vi "GetCntrlRefs.vi"(11 "CntrlRefs":T1) -> (3 "CntrlRefs":T1)   [LabVIEW 2018]
uses:
  CntrlRefs.ctl
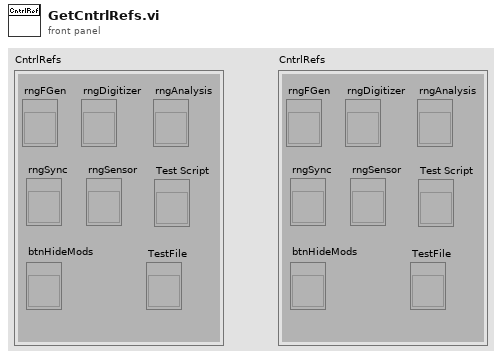
[diagram p1: front panel]
types:
  T1 = typedef "CntrlRefs.ctl" = cluster{"rngFGen":refnum<vi>, "rngDigitizer":refnum<vi>, "rngAnalysis":refnum<vi>, "rngSync":refnum<vi>, "btnHideMods":refnum<vi>, "rngSensor":refnum<vi>, "Test Script":refnum<vi>, "TestFile":refnum<vi>}
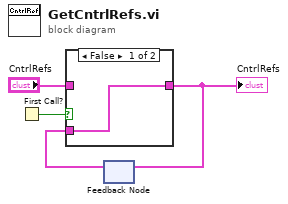
[diagram p0: block diagram]
diagram:
  n1 = First Call?() -> (First Call?: T/F=w4:bool)
  n2 = feedback #1() -> (w1:T1)  [unwired: 1 in]
  n3 = case shown="False" w4 {
    tunnel: "CntrlRefs" -> [_ w6]
    tunnel: [w5 w6] -> w2
    tunnel: w1 -> [w5 _]
    frame False {
    }
    frame True {
    }
  }
  "CntrlRefs" <- w2
  n4 = feedback-in #1(w2) -> ()
